vi "Receive Command.vi"(10 "Consumer Queues":T1, 11 "DAC Process Command in":refnum<class "Generic DAC Process Command.lvclass">) -> (0 "error out":errorcluster, 3 "Generic Command out":refnum<class "Generic Command.lvclass">)   [LabVIEW 2019, in "DAC Process.lvlib" / "Generic DAC Process Command.lvclass"]
uses:
  Generic DAC Process Command.lvclass
  TS Framework/Consumer Queues.ctl
  UI Process/Generic UI Command/Generic UI Process Command.lvclass
  C:/Users/krio/Documents/LV_Projects/TestStand/App/Generic Command/Generic Command.lvclass
  Trig Process/Generic Trig Command/Generic Trig Process Command.lvclass
  Generic Command/Generic Command.lvclass
  TS Framework/TS Framework.lvlib
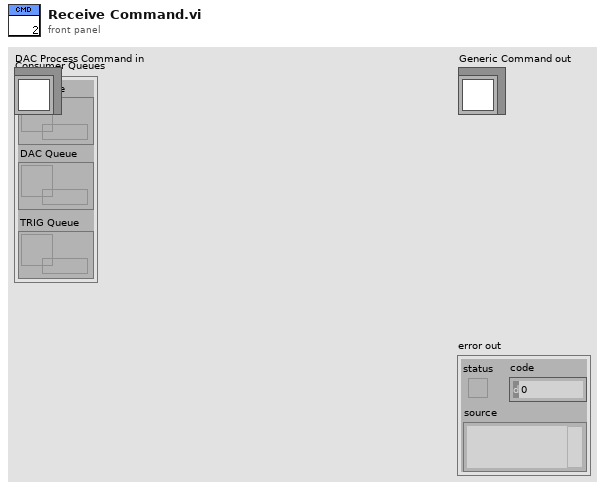
[diagram p1: front panel]
types:
  T1 = typedef "TS Framework.lvlib/Consumer Queues.ctl" = cluster{"UI Queue":refnum<queue>, "DAC Queue":refnum<queue>, "TRIG Queue":refnum<queue>}
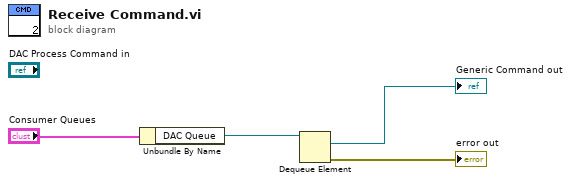
[diagram p0: block diagram]
diagram:
  n1 = Unbundle By Name("Consumer Queues") -> ("DAC Queue"=w3:refnum<queue>)
  n2 = Dequeue Element(queue=w3) -> (element=→"Generic Command out":refnum<class "Generic DAC Process Command.lvclass">, error out=→"error out":errorcluster)  [unwired: 2 in, 2 out]
